vi "Create Excel from Hidden.vi"(0 "DataFilePath":path, 7 "TemplatePath":path, 11 "CMD Step":dbl format="%#_13g") -> (4 "Stat_Path":path, 6 "Data_Path":path, 8 "Spec_Path":path, 15 "Error Out":errorcluster)   [LabVIEW 2013]
uses:
  <vilib>/Utility/file.llb/Read From Spreadsheet File (string).vi
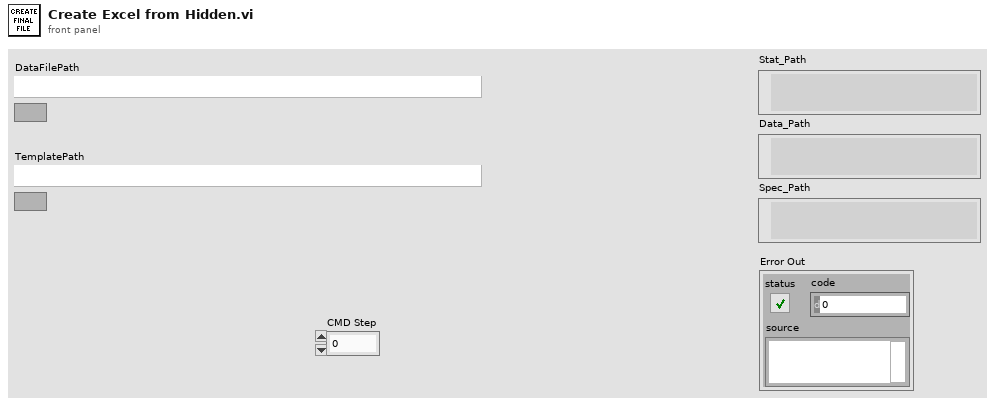
[diagram p1: front panel]
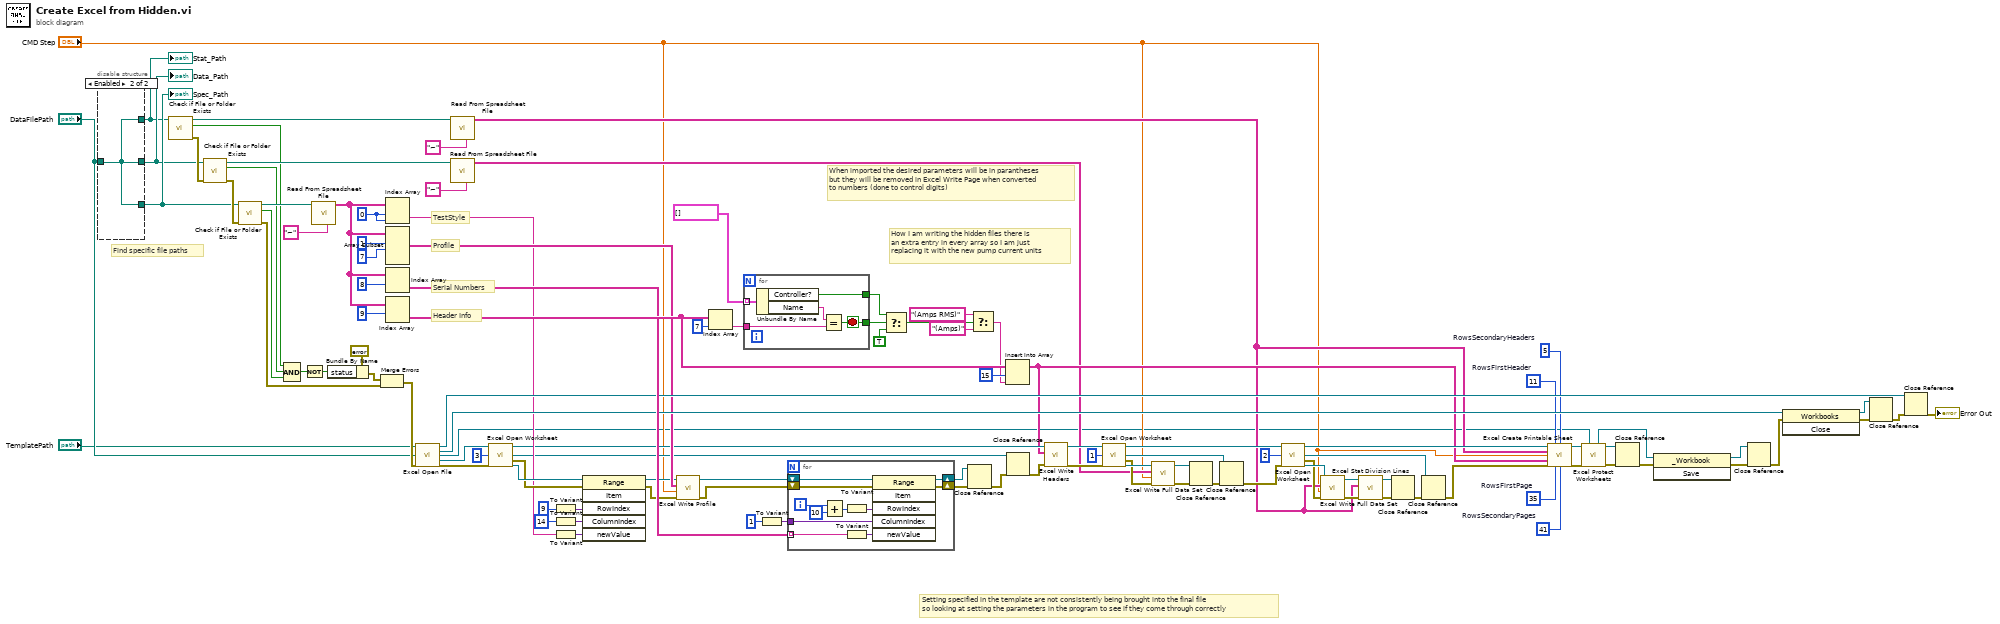
[diagram p0: block diagram]
diagram:
  w16 = 41  # RowsSecondaryPages
  w17 = 35  # RowsFirstPage
  w18 = 5  # RowsSecondaryHeaders
  w19 = 11  # RowsFirstHeader
  w80 = 0 ("index (row)")
  # "Find specific file paths"
  # "Setting specified in the template are not consistently being brought into the final file\nso looking at setting the parameters in the program to see if they come through correctly"
  # "When imported the desired parameters will be in parantheses\nbut they will be removed in Excel Write Page when converted\nto numbers (done to control digits)"
  # "How I am writing the hidden files there is\nan extra entry in every array so I am just\nreplacing it with the new pump current units"
  # "Header Info"
  # "Serial Numbers"
  # "Profile"
  # "TestStyle"
  n1 = disable-structure shown="Enabled" {
    disable-tunnel: [w112 w113] -> w87
    disable-tunnel: [w112 w113] -> w86
    disable-tunnel: [w112 w113] -> w85
    disable-tunnel: "DataFilePath" -> [w112 w113]
    frame Disabled {
    }
    frame Enabled {
    }
  }
  "Stat_Path" <- w85
  "Data_Path" <- w86
  "Spec_Path" <- w87
  n2 = call <vilib>:"Check if File or Folder Exists.vi"("path"=w85) -> ("error out"=w96:errorcluster, "file or folder exists?"=w93:bool, "dup path"=w98:path)  [unwired: 8 in]
  n3 = call <vilib>:"Check if File or Folder Exists.vi"("error in (no error)"=w96, "path"=w86) -> ("error out"=w97:errorcluster, "file or folder exists?"=w94:bool, "dup path"=w100:path)  [unwired: 7 in]
  n4 = call <vilib>:"Check if File or Folder Exists.vi"("error in (no error)"=w97, "path"=w87) -> ("error out"=w43:errorcluster, "file or folder exists?"=w95:bool, "dup path"=w99:path)  [unwired: 7 in]
  n5 = Compound Arithmetic op=AND(w93, w94, w95) -> (w92:bool)
  n6 = Not(x=w92) -> (.not. x?=w90:bool)
  n7 = call-poly <vilib>:"Read From Spreadsheet File.vi"("delimiter (\\t)"="~" ("delimiter (\\t)"), "file path (dialog if empty)"=w99) -> ("all rows"=w108:string[][])  [unwired: 5 in, 4 out]
  n8 = Bundle By Name(cluster=errorcluster {"status"=FALSE, "code"=0, "source"=""} ("error constant"), "status"=w90) -> (w89:errorcluster)
  n9 = Merge Errors(w89, w43) -> (w42:errorcluster)
  n10 = Index Array(array=w108, index (row)=w80, index (col)=w80) -> (element=w33:string)
  n11 = Array Subset(array=w108, index (row)=1 ("index"), length (row)=7 ("length")) -> (w35:string[][])  [unwired: 2 in]
  n12 = Index Array(array=w108, index (row)=8) -> (element=w68:string[])  [unwired: 1 in]
  n13 = Index Array(array=w108, index (row)=9) -> (element=w71:string[])  [unwired: 1 in]
  n14 = call "Excel Open File.vi"("TemplatePath"="TemplatePath", "DataFilePath"="DataFilePath", "Error In"=w42) -> ("Excel Ref Out"=w41:refnum<k7>, "WorkbookS Ref Out"=w40:refnum<k7>, "Workbook Ref Out"=w3:refnum<k7>, "Sheets Ref Out"=w39:refnum<k7>, "Error Out"=w38:errorcluster)  [unwired: 8 in]
  n15 = call-poly <vilib>:"Read From Spreadsheet File.vi"("delimiter (\\t)"="~" ("delimiter (\\t)"), "file path (dialog if empty)"=w98) -> ("all rows"=w15:string[][])  [unwired: 5 in, 4 out]
  n16 = call-poly <vilib>:"Read From Spreadsheet File.vi"("delimiter (\\t)"="~" ("delimiter (\\t)"), "file path (dialog if empty)"=w100) -> ("all rows"=w14:string[][])  [unwired: 5 in, 4 out]
  n17 = call "Excel Open Worksheet.vi"("Sheets Ref In"=w39, "Sheet#"=3, "Error In"=w38) -> ("Sheets Ref Out"=w32:refnum<k7>, "Worksheet Ref Out"=w31:refnum<k7>, "Error Out"=w36:errorcluster, "Cells Ref Out"=w37:refnum<k7>)  [unwired: 9 in]
  n18 = To Variant(anything=9) -> (Variant=w84:variant)
  n19 = To Variant(anything=14) -> (Variant=w81:variant)
  n20 = To Variant(anything=w33) -> (Variant=w82:variant)
  n21 = invoke class="Range" method="Item"(reference=w37, error in=w36, "RowIndex"=w84, "ColumnIndex"=w81, "newValue"=w82) -> (reference out=w13:refnum<k7>, error out=w34:errorcluster)  [unwired: 1 in, 4 out]
  n22 = call "Excel Write Profile.vi"("Error In"=w34, "CMD Step"="CMD Step", "Profile"=w35, "Cells Ref In"=w13) -> ("Error Out"=w30:errorcluster, "Cells Ref Out"=w29:refnum<k7>)  [unwired: 6 in]
  n23 = Index Array(array=w71, index=7) -> (element=w78:string)
  n24 = for {
    tunnel: cluster{"Controller?":bool, "Name":string}[] [] -> [w118] mode=indexing
    tunnel: w78 -> [w116]
    tunnel: [w115] -> w77
    tunnel: [w114] -> w73
    stop <- w114 stop-if-true
    n25 = Unbundle By Name(w118) -> ("Controller?"=w115:bool, "Name"=w117:string)
    n26 = Equal?(x=w117, y=w116) -> (x = y?=w114:bool)
  }
  n27 = To Variant(anything=1 ("y")) -> (Variant=w101:variant)
  n28 = for {
    tunnel: w68 -> [w126] mode=indexing
    tunnel: w101 -> [w122]
    shift-right: [w120] -> w67
    shift-left: w29 -> [w127]
    shift-right: [w119] -> w66
    shift-left: w30 -> [w121]
    i -> [w124]
    n29 = Add(x=w124, y=10) -> (x+y=w123:i32)
    n30 = To Variant(anything=w123) -> (Variant=w129:variant)
    n31 = To Variant(anything=w126) -> (Variant=w128:variant)
    n32 = invoke class="Range" method="Item"(reference=w127, error in=w121, "RowIndex"=w129, "ColumnIndex"=w122, "newValue"=w128) -> (reference out=w120:refnum<k7>, error out=w119:errorcluster)  [unwired: 1 in, 4 out]
  }
  n33 = Select(t=w77, s=w73, f=TRUE) -> (s? t:f=w72:bool)
  n34 = Close Reference(reference=w67, error in (no error)=w66) -> (error out=w62:errorcluster)
  n35 = Select(t="(Amps RMS)", s=w72, f="(Amps)") -> (s? t:f=w69:string)
  n36 = Insert Into Array(array=w71, index=15, new element=w69) -> (w20:string[])
  n37 = Close Reference(reference=w31, error in (no error)=w62) -> (error out=w45:errorcluster)
  n38 = call "Excel Write Headers.vi"("Error In"=w45, "Header Info"=w20, "Sheets Ref In"=w32) -> ("Error Out"=w27:errorcluster, "Sheets Ref Out"=w28:refnum<k7>)  [unwired: 7 in]
  n39 = call "Excel Open Worksheet.vi"("Sheets Ref In"=w28, "Sheet#"=1, "Error In"=w27) -> ("Sheets Ref Out"=w48:refnum<k7>, "Worksheet Ref Out"=w52:refnum<k7>, "Error Out"=w53:errorcluster, "Cells Ref Out"=w54:refnum<k7>)  [unwired: 9 in]
  n40 = call "Excel Write Full Data Set.vi"("Error In"=w53, "CMD Step"="CMD Step", "Data In"=w14, "Cells Ref In"=w54) -> ("Error Out"=w61:errorcluster, "Cells Ref Out"=w60:refnum<k7>)  [unwired: 6 in]
  n41 = Close Reference(reference=w60, error in (no error)=w61) -> (error out=w63:errorcluster)
  n42 = Close Reference(reference=w52, error in (no error)=w63) -> (error out=w47:errorcluster)
  n43 = call "Excel Open Worksheet.vi"("Sheets Ref In"=w48, "Sheet#"=2, "Error In"=w47) -> ("Sheets Ref Out"=w26:refnum<k7>, "Worksheet Ref Out"=w49:refnum<k7>, "Error Out"=w50:errorcluster, "Cells Ref Out"=w51:refnum<k7>)  [unwired: 9 in]
  n44 = call "Excel Write Full Data Set.vi"("Error In"=w50, "CMD Step"="CMD Step", "Data In"=w15, "Cells Ref In"=w51) -> ("Error Out"=w56:errorcluster, "Cells Ref Out"=w57:refnum<k7>)  [unwired: 6 in]
  n45 = call "Excel Stat Division Lines.vi"("Error In"=w56, "Data In"=w15, "Cells Ref In"=w57) -> ("Error Out"=w58:errorcluster, "Cells Ref Out"=w59:refnum<k7>)  [unwired: 7 in]
  n46 = Close Reference(reference=w59, error in (no error)=w58) -> (error out=w64:errorcluster)
  n47 = Close Reference(reference=w49, error in (no error)=w64) -> (error out=w25:errorcluster)
  n48 = call "Excel Create Printable Sheet.vi"("Sheets Ref In"=w26, "RowsFirstHeader"=w19, "RowsHeadersAfter"=w18, "Stat Array"=w15, "CMD Step"="CMD Step", "HeaderInfo"=w20, "Error In"=w25, "RowsFirstPage"=w17, "RowsPagesAfter"=w16) -> ("Sheets Ref Out"=w24:refnum<k7>, "Error Out"=w23:errorcluster)  [unwired: 5 in]
  n49 = call "Excel Protect Worksheets.vi"("Sheets Ref In"=w24, "Workbook Ref In"=w3, "Error In"=w23) -> ("Workbook Ref Out"=w2:refnum<k7>, "Sheets Ref Out"=w22:refnum<k7>, "Error Out"=w21:errorcluster)  [unwired: 10 in]
  n50 = Close Reference(reference=w22, error in (no error)=w21) -> (error out=w65:errorcluster)
  n51 = invoke class="_Workbook" method="Save"(reference=w2, error in=w65) -> (reference out=w7:refnum<k7>, error out=w10:errorcluster)  [unwired: 1 in, 1 out]
  n52 = Close Reference(reference=w7, error in (no error)=w10) -> (error out=w9:errorcluster)
  n53 = invoke class="Workbooks" method="Close"(reference=w40, error in=w9) -> (reference out=w8:refnum<k7>, error out=w11:errorcluster)  [unwired: 1 in, 1 out]
  n54 = Close Reference(reference=w8, error in (no error)=w11) -> (error out=w12:errorcluster)
  n55 = Close Reference(reference=w41, error in (no error)=w12) -> (error out=→"Error Out":errorcluster)
